vi "write_signal_hdf5.vi"(7 "Index":i32, 8 "error in":errorcluster, 10 "Save Path":path, 11 "Signal array":T2[](array[typedef])) -> (0 "error out":errorcluster, 3 "Signal Processing:":T4={"Integer Timestamp"=0, "Dust Event ID"=0, "Role ID"=enum."First_Detector", "Data"=[], "Signal Length"=0, "dt"=0.0, "Offset"=0.0, "Hardware ID"=enum."CSA 1"})   [LabVIEW 2013]
uses:
  Public API/Post_Signal.ctl
  Controls/Role ID.ctl
  Controls/Hardware ID.ctl
  Public API/Signal.ctl
  <vilib>/addons/h5labview/polymorph/H5D_write_var.vi
  <vilib>/addons/h5labview/H5Dataset.lvlib
  <vilib>/addons/h5labview/H5Attrib.lvlib
panel:
  out "concatenated string":string
  out "Role ID":T1
  # "Signal"
  # "Signal"
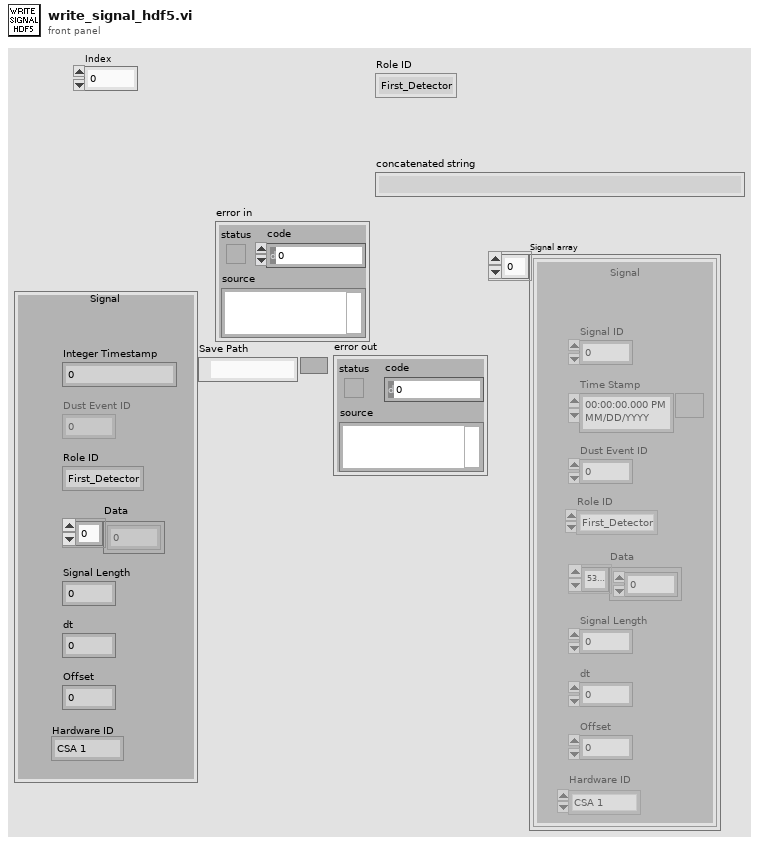
[diagram p1: front panel]
types:
  T1 = typedef "Role ID.ctl" = enum16{"First_Detector", "Second_Detector", "Third_Detector", "LeCroy_CH1", "LeCroy_CH2", "LeCroy_CH3", "LeCroy_CH4", "PSU"}
  T2 = typedef "Signal.ctl" = cluster{"Signal ID":i64, "Time Stamp":timestamp, "Dust Event ID":i64, "Role ID":T1, "Data":sgl[], "Signal Length":i32, "dt":sgl, "Offset":dbl, "Hardware ID":T3}
  T3 = typedef "Hardware ID.ctl" = enum16{"Unknown", "CSA 1", "CSA 2", "CSA 3", "CSA 4", "CSA 5", "CSA 6"}
  T4 = typedef "Post_Signal.ctl" = cluster{"Integer Timestamp":i64, "Dust Event ID":i64, "Role ID":T1, "Data":sgl[], "Signal Length":i32, "dt":sgl, "Offset":dbl, "Hardware ID":T3}
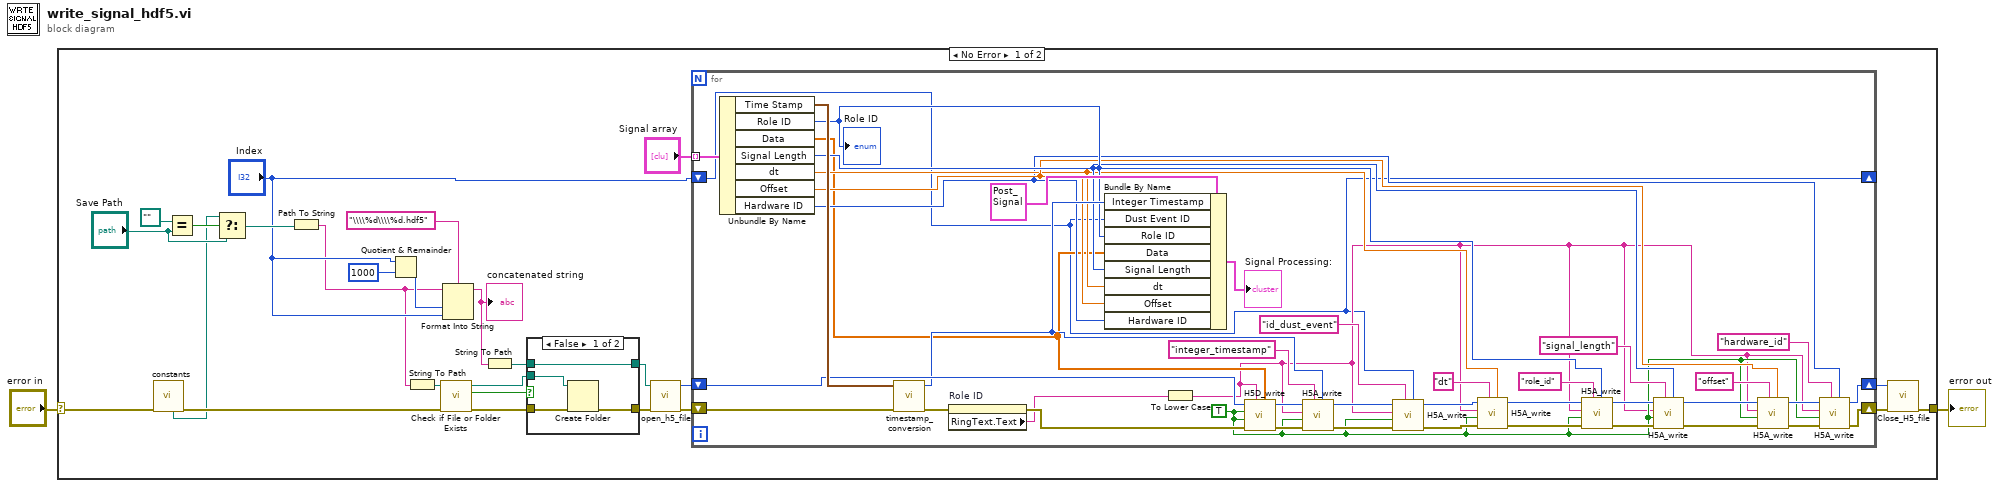
[diagram p0: block diagram]
diagram:
  n1 = case shown="No Error" "error in" {
    selector: "error in" -> [w22 w77]
    tunnel: [w23 w77] -> w1
    frame No Error {
      n2 = call "constants.vi"("error in (no error)"=w22) -> ("error out"=w14:errorcluster, "file path for Processed Signal .hdf5 files"=w9:path)  [unwired: 4 in, 5 out]
      n3 = Equal?(x=path "" ("Save Path"), y="Save Path") -> (x = y?=w19:bool)
      n4 = Select(t=w9, s=w19, f="Save Path") -> (s? t:f=w21:path)
      n5 = Path To String(path=w21) -> (string=w3:string)
      n6 = Quotient & Remainder(x="Index", y=1000) -> (floor(x/y)=w4:i32)  [unwired: 1 out]
      n7 = String To Path(string=w3) -> (path=w13:path)
      n8 = call <vilib>:"Check if File or Folder Exists.vi"("error in (no error)"=w14, "path"=w13) -> ("error out"=w15:errorcluster, "file or folder exists?"=w17:bool, "dup path"=w16:path)  [unwired: 7 in]
      n9 = Format Into String(format string="\\\\%d\\\\%d.hdf5", initial string=w3, w4, "Index") -> (resulting string=w6:string)  [unwired: 1 in, 1 out]
      "concatenated string" <- w6
      n10 = String To Path(string=w6) -> (path=w11:path)
      n11 = case shown="False" w17 {
        tunnel: w16 -> [w32 _]
        tunnel: w15 -> [w31 w34]
        tunnel: [w30 w34] -> w12
        tunnel: w11 -> [w29 w33]
        tunnel: [w29 w33] -> w10
        frame False {
          n12 = Create Folder(path (use dialog)=w32, error in=w31) -> (error out=w30:errorcluster)  [unwired: 1 in, 2 out]
        }
        frame True {
        }
      }
      n13 = call "open_h5_file.vi"("error in (no error)"=w12, "path"=w10) -> ("error out"=w27:errorcluster, "ref"=w26:i32)  [unwired: 8 in]
      n14 = for {
        tunnel: "Signal array" -> [w74] mode=indexing
        shift-right: [w48] -> w24
        shift-left: w27 -> [w73]
        shift-right: [w35] -> _
        shift-left: "Index" -> [w35]
        shift-right: [w47] -> w25
        shift-left: w26 -> [w70]
        w40 = TRUE ("preserve attribs?")
        n15 = Unbundle By Name(w74) -> ("Time Stamp"=w75:timestamp, "Role ID"=w59:T1, "Data"=w38:sgl[], "Signal Length"=w58:i32, "dt"=w41:sgl, "Offset"=w57:dbl, "Hardware ID"=w39:T3)
        "Role ID" <- w59
        n16 = call "timestamp_conversion.vi"("error in (no error)"=w73, "Time Stamp"=w75) -> ("error out"=w71:errorcluster, "Integer Time"=w65:i64)  [unwired: 7 in]
        n17 = property on="Role ID" class="Enum (strict)"(error in=w71) -> (error out=w69:errorcluster, "RingText.Text"=w37:string)  [unwired: 1 in, 1 out]
        n18 = Bundle By Name(cluster=T4 {"Integer Timestamp"=0, "Dust Event ID"=0, "Role ID"=enum."First_Detector", "Data"=[], "Signal Length"=0, "dt"=0.0, "Offset"=0.0, "Hardware ID"=enum."CSA 1"} ("Post_Signal 2"), "Integer Timestamp"=w65, "Dust Event ID"=w35, "Role ID"=w59, "Data"=w38, "Signal Length"=w58, "dt"=w41, "Offset"=w57, "Hardware ID"=w39) -> (→"Signal Processing:":T4)
        n19 = To Lower Case(string=w37) -> (all lower case string=w36:string)
        n20 = call-poly <vilib>:"H5D_write.vi"("data"=w38, "name"=w36, "error in (no error)"=w69, "overwrite?"=w40, "preserve attribs?"=w40, "ref"=w70) -> ("error out"=w67:errorcluster, "ref out"=w68:i32)  [unwired: 2 in]
        n21 = call <vilib>:"H5A_write.vi"("value"=w65, "attrib_name"="integer_timestamp", "error in (no error)"=w67, "overwrite? (F)"=w40, "obj_name"=w36, "ref"=w68) -> ("error out"=w53:errorcluster, "ref out"=w52:i32)  [unwired: 2 in]
        n22 = call <vilib>:"H5A_write.vi"("value"=w35, "attrib_name"="id_dust_event", "error in (no error)"=w53, "overwrite? (F)"=w40, "obj_name"=w36, "ref"=w52) -> ("error out"=w46:errorcluster, "ref out"=w43:i32)  [unwired: 2 in]
        n23 = call <vilib>:"H5A_write.vi"("value"=w41, "attrib_name"="dt", "error in (no error)"=w46, "overwrite? (F)"=w40, "obj_name"=w36, "ref"=w43) -> ("error out"=w45:errorcluster, "ref out"=w42:i32)  [unwired: 2 in]
        n24 = call <vilib>:"H5A_write.vi"("value"=w59, "attrib_name"="role_id", "error in (no error)"=w45, "overwrite? (F)"=w40, "obj_name"=w36, "ref"=w42) -> ("error out"=w54:errorcluster, "ref out"=w49:i32)  [unwired: 2 in]
        n25 = call <vilib>:"H5A_write.vi"("value"=w58, "attrib_name"="signal_length", "error in (no error)"=w54, "overwrite? (F)"=w40, "obj_name"=w36, "ref"=w49) -> ("error out"=w55:errorcluster, "ref out"=w50:i32)  [unwired: 2 in]
        n26 = call <vilib>:"H5A_write.vi"("value"=w57, "attrib_name"="offset", "error in (no error)"=w55, "overwrite? (F)"=w40, "obj_name"=w36, "ref"=w50) -> ("error out"=w56:errorcluster, "ref out"=w51:i32)  [unwired: 2 in]
        n27 = call <vilib>:"H5A_write.vi"("value"=w39, "attrib_name"="hardware_id", "error in (no error)"=w56, "overwrite? (F)"=w40, "obj_name"=w36, "ref"=w51) -> ("error out"=w48:errorcluster, "ref out"=w47:i32)  [unwired: 2 in]
      }
      n28 = call "Close_H5_file.vi"("error in (no error)"=w24, "ref"=w25) -> ("error out"=w23:errorcluster)  [unwired: 9 in]
    }
    frame Error {
    }
  }
  "error out" <- w1
